vi "Write Target Angle.vi"(11 "Detected Targets":T2(array[cluster])) -> ()   [LabVIEW 2015]
uses:
  vision/Camera Types.ctl
  <vilib>/Rock Robotics/Network Tables/NT Write Number.vi
panel:
  in  "Camera Type":T1
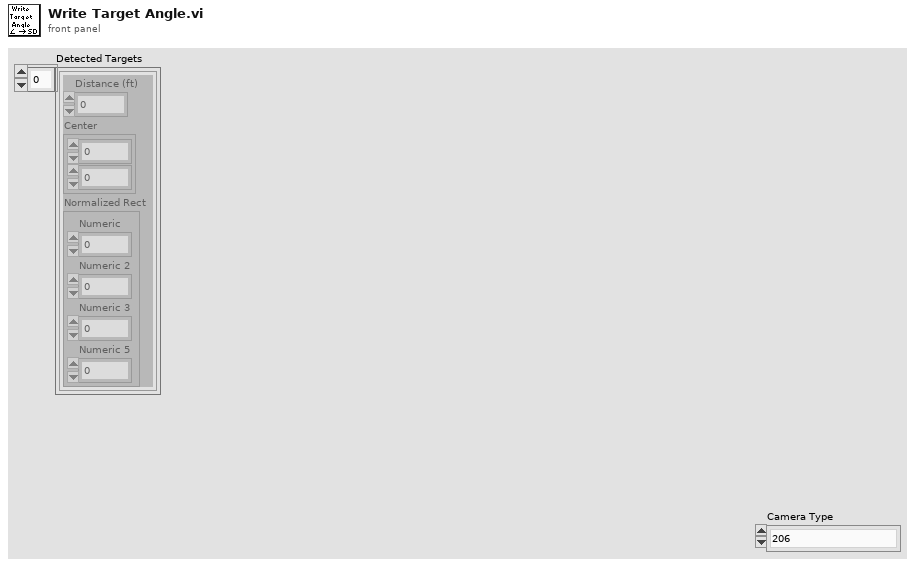
[diagram p1: front panel]
types:
  T1 = typedef "Camera Types.ctl" = enum16{"206", "1011", "1013", "MS HD3000 square", "MS HD3000 640x480"}
  T2 = cluster{"Distance (ft)":dbl, "Center":cluster{dbl, dbl}, "Normalized Rect":cluster{"Numeric":dbl, "Numeric 2":dbl, "Numeric 3":dbl, "Numeric 5":dbl}}[]
  T3 = cluster{"Distance (ft)":dbl, "Center":cluster{dbl, dbl}, "Normalized Rect":cluster{"Numeric":dbl, "Numeric 2":dbl, "Numeric 3":dbl, "Numeric 5":dbl}}
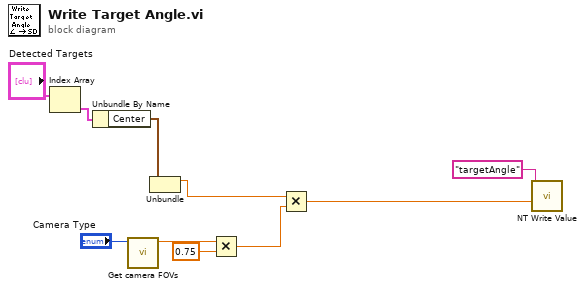
[diagram p0: block diagram]
diagram:
  n1 = Index Array(array="Detected Targets") -> (element=w9:T3)  [unwired: 1 in]
  n2 = Unbundle By Name(w9) -> ("Center"=w10:cluster{dbl, dbl})
  n3 = call "Get camera FOVs.vi"("Camera Type"="Camera Type") -> ("FOV"=w5:dbl)  [unwired: 9 in, 1 out]
  n4 = Unbundle(w10) -> (w3:dbl)  [unwired: 1 out]
  n5 = Multiply(x=w5, y=0.75) -> (x*y=w2:dbl)
  n6 = Multiply(x=w3, y=w2) -> (x*y=w1:dbl)
  n7 = call-poly <vilib>:"NT Write Value.vi"("Numeric"=w1, "Name"="targetAngle") -> ()  [unwired: 9 in, 1 out]
